vi "Get Iteration Time Collision.vi"(7 "Movable in":refnum<class "Movable.lvclass">, 11 "Collision in":refnum<class "Collision.lvclass">) -> (2 "Time factor out":dbl format="%#_13g")   [LabVIEW 2024, in "Collision.lvclass"]
doc: "MIT Licence\nCopyright (c) 2024 David Grollier"
uses:
  Collision.lvclass
  Game Componants/Game Board Component/Movable/Movable.lvclass
  Collision.lvclass/Collision.ctl
  Game Componants/Game Board Component/Movable/Movable.lvclass/Movable.ctl
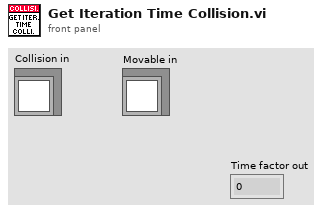
[diagram p1: front panel]
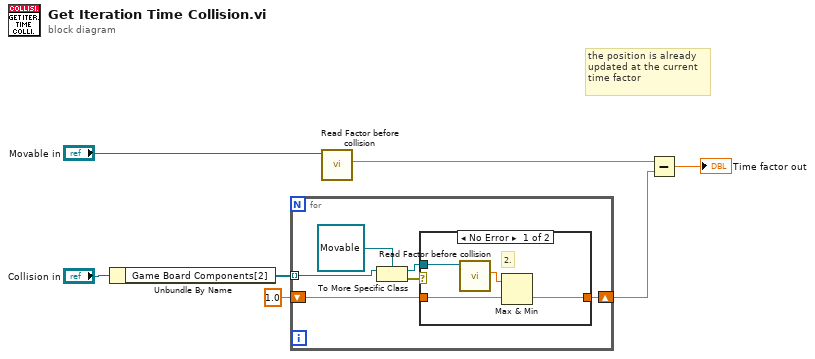
[diagram p0: block diagram]
diagram:
  # "the position is already updated at the current time factor"
  n1 = Unbundle By Name("Collision in") -> ("Game Board Components[2]"=w6:refnum<class "Game Board Component.lvclass">[])
  n2 = for {
    tunnel: w6 -> [w12] mode=indexing
    shift-right: [w9] -> w2
    shift-left: 1.0 -> [w10]
    n3 = To More Specific Class(target class=refnum<class "Movable.lvclass"> refnum ("Movable.lvclass"), reference=w12) -> (specific class reference=w11:refnum<class "Movable.lvclass">, error out=w8:errorcluster)  [unwired: 1 in]
    n4 = case shown="No Error" w8 {
      tunnel: w11 -> [w16 _]
      tunnel: w10 -> [w17 w18]
      tunnel: [w14 w18] -> w9
      frame No Error {
        # "2."
        n5 = call "Read Factor before collision.vi"("Movable in"=w16) -> ("Factor before collision"=w15:dbl)  [unwired: 10 in]
        n6 = Max & Min(x=w15, y=w17) -> (min(x,y)=w14:dbl)  [unwired: 1 out]
      }
      frame Error {
        # "Not a movable : doesn't move"
      }
    }
  }
  n7 = call "Read Factor before collision.vi"("Movable in"="Movable in") -> ("Factor before collision"=w3:dbl)  [unwired: 10 in]
  n8 = Subtract(x=w3, y=w2) -> (x-y=→"Time factor out":dbl)
